vi "Read DeviceType.vi"(8 "error in (no error)":errorcluster, 11 "CCD in":refnum<class "CCD.lvclass">) -> (0 "error out":errorcluster, 2 "device type":string, 3 "CCD out":refnum<class "CCD.lvclass">)   [LabVIEW 2023, in "CCD.lvclass"]
uses:
  CCD.lvclass
  GenericDevice/GenericDevice.lvclass
  CCD.lvclass/CCD.ctl
panel:
  # "Connector Pane"
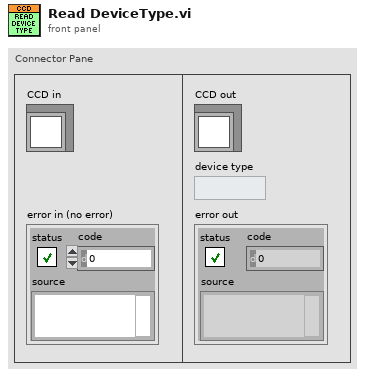
[diagram p1: front panel]
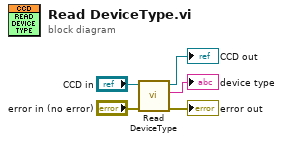
[diagram p0: block diagram]
diagram:
  n1 = call-parent "Read DeviceType.vi"("error in (no error)"="error in (no error)", "GenericDevice in"="CCD in") -> ("error out"=→"error out":errorcluster, "device type"=→"device type":string, "GenericDevice out"=→"CCD out":refnum<class "CCD.lvclass">)  [unwired: 7 in]
